vi "QC_RunInformation.vi"() -> ()   [LabVIEW 2013]
panel:
  out "LocalConfiguration":T1={"Institute"="", "Manufacturers"=[], "Devices"=[], "Serialnumbers Lookup DB"="", "Data directory"="", "Backup & screenshot directory"="", "List of known users"=[], "Measurement switch not used"=TRUE, "Measurement Switch"="Pickering Matrix", "DUT Switch"="Keithley 3706A", "Rseries IV [MOhm]"="", "Rshunt IV [MOhm]"="", "Rseries CV [MOhm]"="", "DC blocking Cap [µF]"="", "Rseries LCR [MOhm]"="", "Rseries stability [MOhm]"="", "Rshunt stability [MOhm]"="", "Rseries striptest bias [MOhm]"="", "Rseries strip pinhole [MOhm]"=""}
  in  "Run info":T2={"Sensor Serial No.:"="", "Wafer:"="", "Batch:"="", "Manufacturer:"="Hamamatsu", "Device Category:"="ATLAS18SS", "Database Serial No.:"="", "Date Initiated:"="", "Time Initiated:"="", "Test"="SENSOR_IV", "Probeplan used:"="", "End of Run comment:"="", "User:"="", "Vbias SMU"="", "LCR"="", "Test SMU"="", "Test DMM"=""}
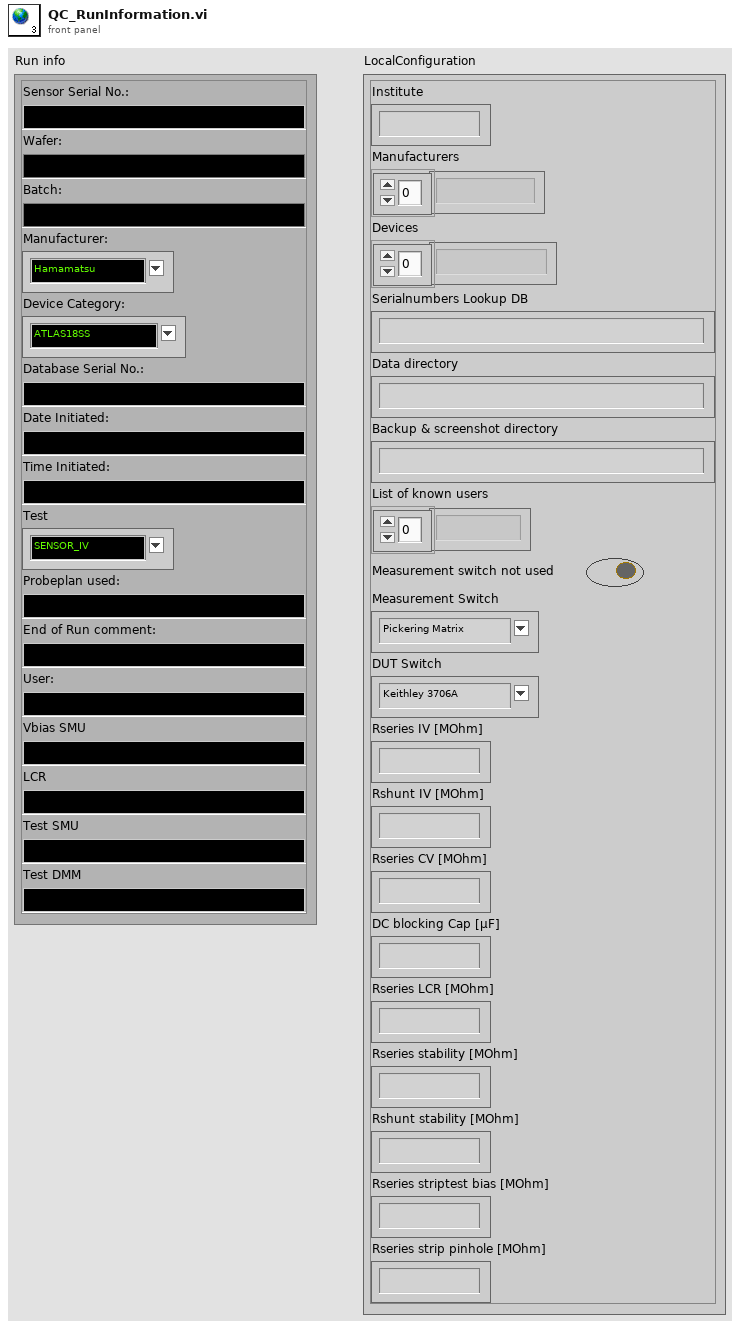
[diagram p1: front panel]
types:
  T1 = cluster{"Institute":string, "Manufacturers":string[], "Devices":string[], "Serialnumbers Lookup DB":string, "Data directory":string, "Backup & screenshot directory":string, "List of known users":string[], "Measurement switch not used":bool, "Measurement Switch":string, "DUT Switch":string, "Rseries IV [MOhm]":string, "Rshunt IV [MOhm]":string, "Rseries CV [MOhm]":string, "DC blocking Cap [µF]":string, "Rseries LCR [MOhm]":string, "Rseries stability [MOhm]":string, "Rshunt stability [MOhm]":string, "Rseries striptest bias [MOhm]":string, "Rseries strip pinhole [MOhm]":string}
  T2 = cluster{"Sensor Serial No.:":string, "Wafer:":string, "Batch:":string, "Manufacturer:":string, "Device Category:":string, "Database Serial No.:":string, "Date Initiated:":string, "Time Initiated:":string, "Test":string, "Probeplan used:":string, "End of Run comment:":string, "User:":string, "Vbias SMU":string, "LCR":string, "Test SMU":string, "Test DMM":string}
diagram:
